vi "Write calibration curves to instruments.vi"(8 "error in (no error)":errorcluster, 11 "LS218 in":refnum<class "LS218.lvclass">) -> (0 "error out":errorcluster, 3 "LS218 out":refnum<class "LS218.lvclass">)   [LabVIEW 2013, in "LS218.lvlib" / "LS218.lvclass"]
doc: "Read calibration curves from file and write to instrument (user calubration 21-28)."
uses:
  LS218.lvclass
  LS218.lvclass/LS218.ctl
  <instrlib>/Lake Shore Cryotronics 218/Lake Shore Cryotronics 218.lvlib
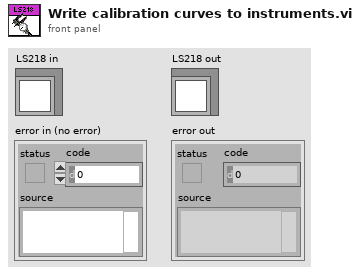
[diagram p1: front panel]
types:
  T1 = cluster{"Index (1)":i32, "Units":dbl, "Temperature":dbl}[]
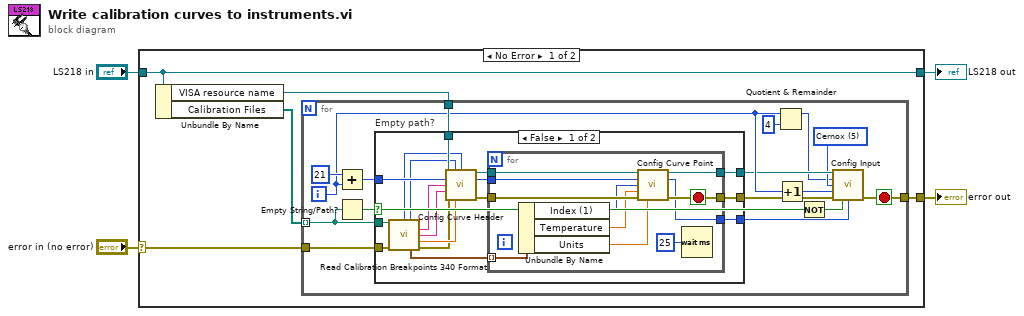
[diagram p0: block diagram]
diagram:
  n1 = case shown="No Error" "error in (no error)" {
    selector: "error in (no error)" -> [w6 w56]
    tunnel: [w5 w56] -> w3
    tunnel: [w9 w55] -> w1
    tunnel: "LS218 in" -> [w9 w55]
    frame No Error {
      n2 = Unbundle By Name(w9) -> ("VISA resource name"=w8:refnum<visa-resource-name>, "Calibration Files"=w7:path[])
      n3 = for {
        tunnel: w8 -> [w24]
        tunnel: w7 -> [w20] mode=indexing
        tunnel: w6 -> [w22]
        tunnel: [w21] -> w5
        i -> [w19]
        stop <- w21 stop-if-true
        w16 = u16 5 items=["2.5V Diode", "7.5V Diode", "250 Ohm Platinum", "500 Ohm Platinum", "5K Ohm Platinum", "Cernox"] ("Sensor Type (0:2.5V Diode)")
        n4 = Add(x=21 ("Curve (21)"), y=w19) -> (x+y=w23:i32)
        n5 = Empty String/Path?(string/path=w20) -> (empty?=w11:bool)
        n6 = case "Empty path?" shown="False" w11 {
          tunnel: w24 -> [w41 w54]
          tunnel: w23 -> [w40 w52]
          tunnel: w22 -> [w39 w53]
          tunnel: w20 -> [w38 _]
          tunnel: [w28 w53] -> w18
          tunnel: [w27 w54] -> w17
          tunnel: [w26 w52] -> w15
          frame False {
            n7 = call "Read Calibration Breakpoints 340 Format.vi"("Calibration File"=w38, "Error In"=w39) -> ("Temp Coefficient"=w32:u16, "Curve Data Format"=w33:u16, "Curve Name"=w35:string, "Curve Serial Number"=w34:string, "Limit Value"=w31:dbl, "Calibration Points"=w29:T1, "Error Out"=w30:errorcluster)  [unwired: 7 in]
            n8 = call <instrlib>:"Config Curve Header.vi"("VISA resource name"=w41, "Curve Data Format (V/K:0)"=w33, "Temp Coefficient (Neg:0)"=w32, "Curve (21)"=w40, "Curve Name (\"\")"=w35, "Curve Serial Number (\"\")"=w34, "error in (no error)"=w30, "Limit Value (475.00)"=w31) -> ("VISA resource name out"=w37:refnum<visa-resource-name>, "error out"=w36:errorcluster)  [unwired: 6 in]
            n9 = for {
              tunnel: w40 -> [w42]
              tunnel: w29 -> [w48] mode=indexing
              tunnel: w37 -> [w51]
              tunnel: w36 -> [w50]
              tunnel: [w49] -> w28
              tunnel: [w43] -> w27
              tunnel: [w42] -> w26
              stop <- w49 stop-if-true
              n10 = Unbundle By Name(w48) -> ("Index (1)"=w47:i32, "Temperature"=w46:dbl, "Units"=w45:dbl)
              n11 = call <instrlib>:"Config Curve Point.vi"("VISA resource name"=w51, "Units Value (0.0000)"=w45, "Curve (21)"=w42, "Index (1)"=w47, "Temperature Value (0.0000)"=w46, "error in (no error)"=w50) -> ("VISA resource name out"=w43:refnum<visa-resource-name>, "error out"=w49:errorcluster)  [unwired: 8 in]
              n12 = Wait (ms)(milliseconds to wait=u32 25) -> ()  [unwired: 1 out]
            }
          }
          frame True {
          }
        }
        n13 = Quotient & Remainder(x=w19, y=4) -> (x-y*floor(x/y)=w13:i32)  [unwired: 1 out]
        n14 = Increment(x=w19) -> (x+1=w14:i32)
        n15 = Not(x=w11) -> (.not. x?=w10:bool)
        n16 = call <instrlib>:"Config Input.vi"("VISA resource name"=w17, "Input Group (0:Inputs 1-4)"=w13, "Sensor Type (0:2.5V Diode)"=w16, "Input (1)"=w14, "error in (no error)"=w18, "Input (T: Input ON)"=w10, "Input Curve (0:None)"=w15) -> ("error out"=w21:errorcluster)  [unwired: 7 in, 1 out]
      }
    }
    frame Error {
    }
  }
  "error out" <- w3
  "LS218 out" <- w1
